vi "Draw_Waveforms.vi"(10 "ODSS Step":dbl[][](array[numeric]), 11 "Comm":dbl) -> (3 "Time M":T1(array[cluster]), 4 "Meter":string[][][](array[string]))   [LabVIEW 2010]
doc: "This VI implements the routine for drawing the votlage waveforms and extracting the informattion porvided by each meter.\n\nCreated by Davis Montenegro\n06-30-2017"
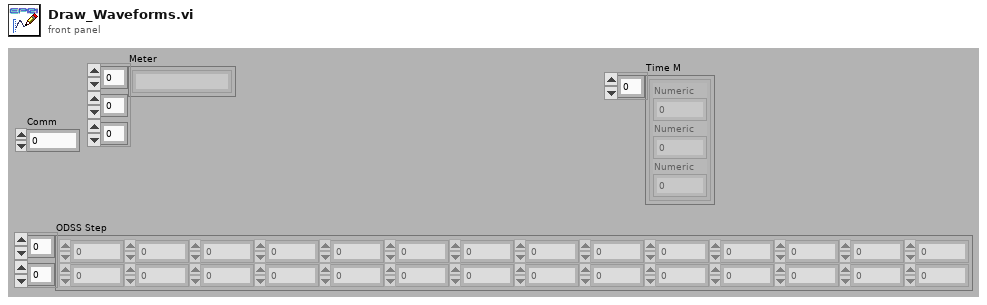
[diagram p1: front panel]
types:
  T1 = cluster{"Numeric":dbl, "Numeric":dbl, "Numeric":dbl}[]
  T2 = cluster{"Numeric":dbl, "Numeric":dbl, "Numeric":dbl}
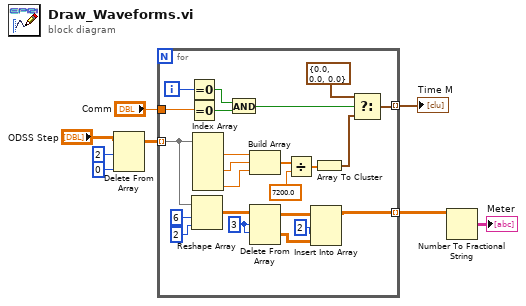
[diagram p0: block diagram]
diagram:
  n1 = Delete From Array(array="ODSS Step", length=2, index (col)=0 ("disabled index (col)")) -> (array with subset deleted=w4:dbl[][])  [unwired: 1 in, 1 out]
  n2 = for {
    tunnel: "Comm" -> [w31]
    tunnel: w4 -> [w24] mode=indexing
    tunnel: [w25] -> w3 mode=indexing
    tunnel: [w9] -> w2 mode=indexing
    i -> [w30]
    w14 = 3 ("length")
    n3 = Equal To 0?(x=w30) -> (x = 0?=w28:bool)
    n4 = Equal To 0?(x=w31) -> (x = 0?=w29:bool)
    n5 = Reshape Array(w24, 6 ("dimension size"), 2 ("dimension size")) -> (w15:dbl[][])
    n6 = Index Array(array=w24) -> (element #1=w21:dbl, element #3=w20:dbl, element #5=w19:dbl)  [unwired: 5 in, 2 out]
    n7 = And(x=w28, y=w29) -> (x .and. y?=w27:bool)
    n8 = Build Array(w21, w20, w19) -> (w18:dbl[])
    n9 = Delete From Array(array=w15, length=w14, index (row)=w14) -> (deleted portion=w11:dbl[][], array with subset deleted=w12:dbl[][])  [unwired: 1 in]
    n10 = Divide(x=w18, y=7200.0) -> (x/y=w17:dbl[])
    n11 = Insert Into Array(array=w12, index (col)=2 ("disabled index (col)"), new element=w11) -> (w9:dbl[][])  [unwired: 1 in]
    n12 = Array To Cluster(array=w17) -> (cluster=w16:cluster{"[0]":dbl, "[1]":dbl, "[2]":dbl})
    n13 = Select(t=T2 {"Numeric"=0.0, "Numeric"=0.0, "Numeric"=0.0}, s=w27, f=w16) -> (s? t:f=w25:cluster{"[0]":dbl, "[1]":dbl, "[2]":dbl})
  }
  "Time M" <- w3
  n14 = Number To Fractional String(number=w2) -> (F-format string=→"Meter":string[][][])  [unwired: 3 in]
